vi "Instrument Manager Loop.vi"(8 "System Control":refnum<queue>, 11 "Instrument Manager":refnum<queue>) -> (0 "error out":errorcluster)   [LabVIEW 2020, in "Mock LC Parser.lvlib" / "Instrument Manager.lvlib"]
uses:
  Instrument Manager.lvlib
  support/Message Queue/Message Cluster.ctl
  Instrument State.ctl
  <vilib>/Utility/error.llb/Error Cluster From Error Code.vi
  <vilib>/ErrorRing/Error Ring.xnode
  support/Message Queue/Message Queue.lvlib
  Mock LC Parser.lvlib
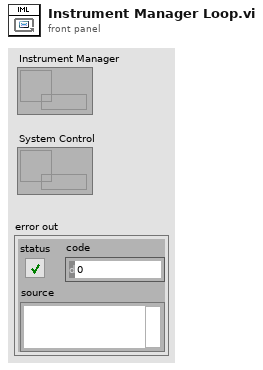
[diagram p1: front panel]
types:
  T1 = cluster{"Time Stamp":timestamp, "Peaks":string[][]}[]
  T2 = typedef "Mock LC Parser.lvlib/Instrument Manager.lvlib/Instrument State.ctl" = cluster{"Data Directory":path, "Last Report Number":i32, "Yield":dbl, "Max Concentration (mM)":dbl, "Report File Pattern":string, "Current Data File":path, "Peak Data Array":cluster{"Time Stamp":timestamp, "Peaks":string[][]}[], "Average Peak Data":cluster{"Time Stamp":timestamp, "Peaks":string[][]}, "Points to Average":i32}
  T3 = cluster{"seconds since 1Jan1904":timestamp, "Peaks":string[][]}
  T4 = cluster{"seconds since 1Jan1904":timestamp, "Peaks":string[][]}[]
  T5 = cluster{"Time Stamp":timestamp, "Peaks":string[][]}
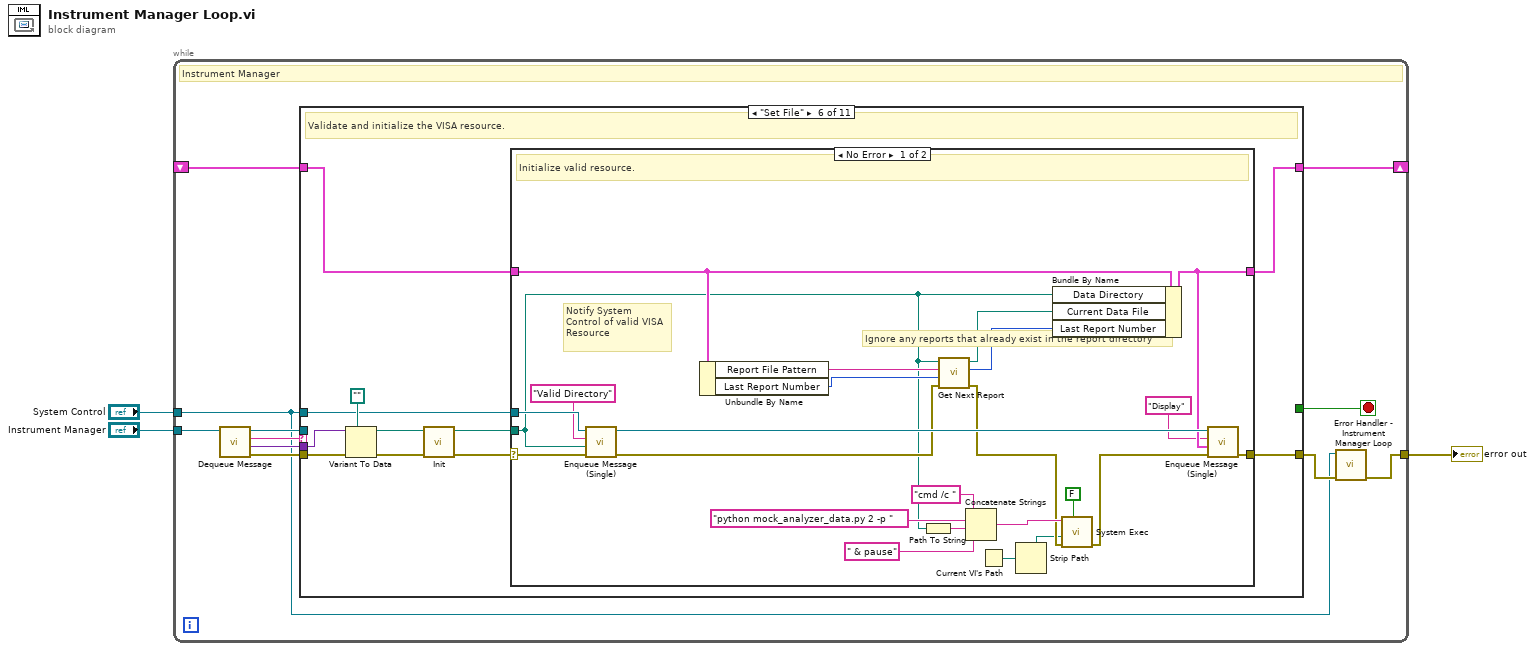
[diagram p0: block diagram]
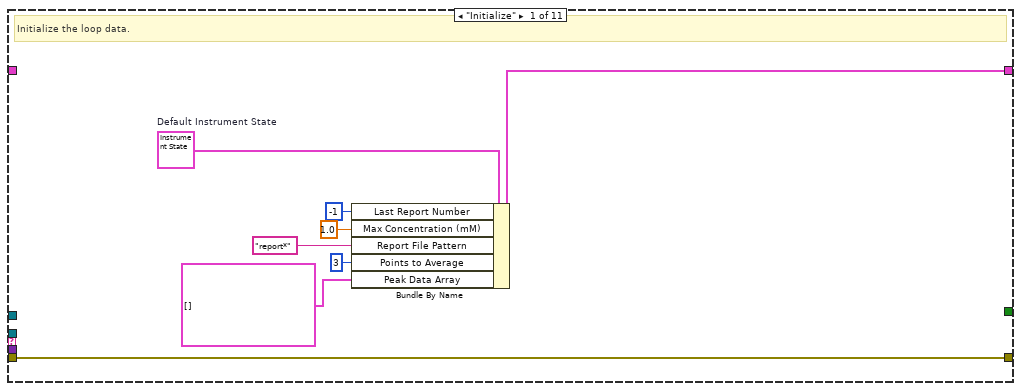
[diagram p2: hidden frame]
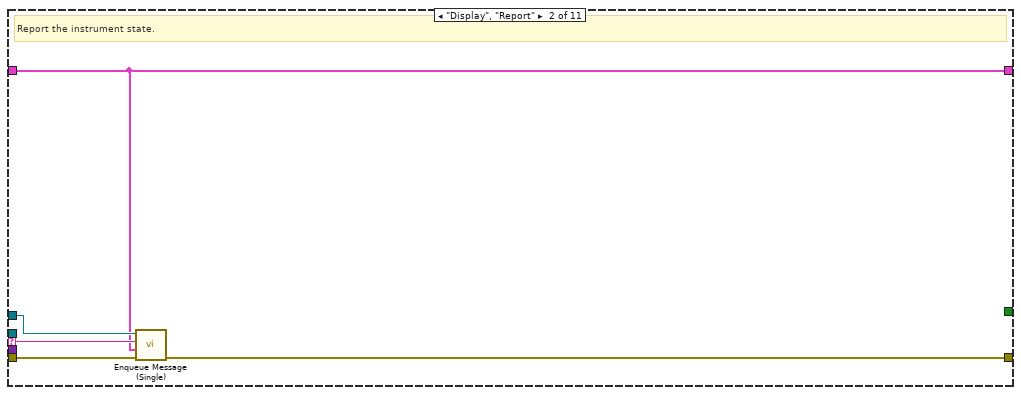
[diagram p3: hidden frame]
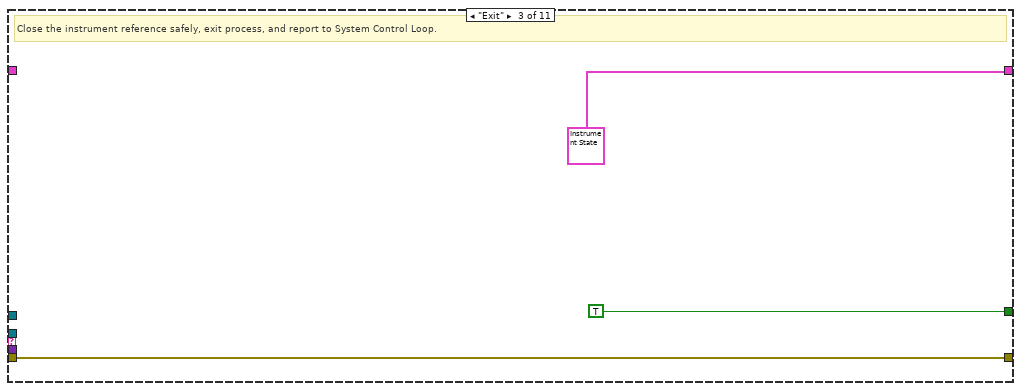
[diagram p4: hidden frame]
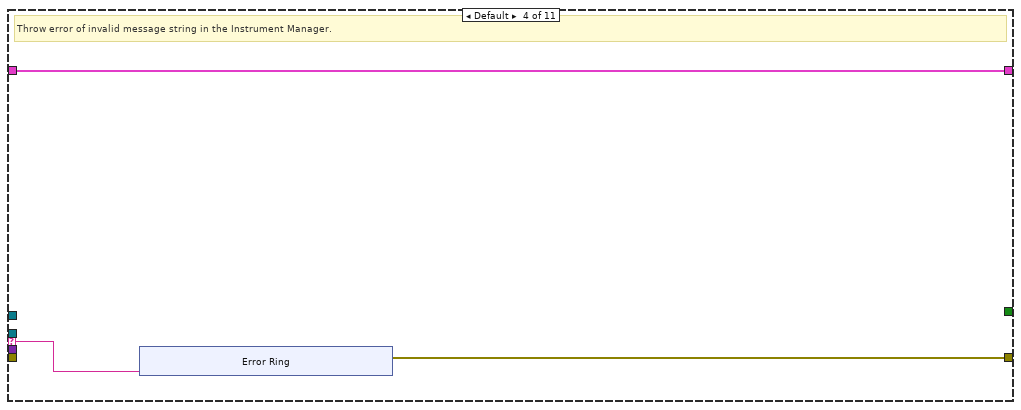
[diagram p5: hidden frame]
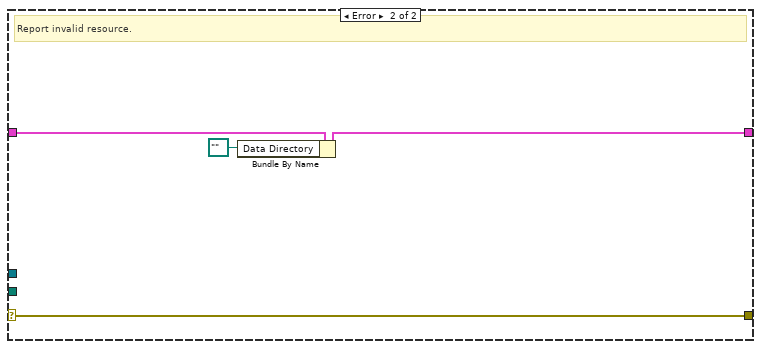
[diagram p7: hidden frame]
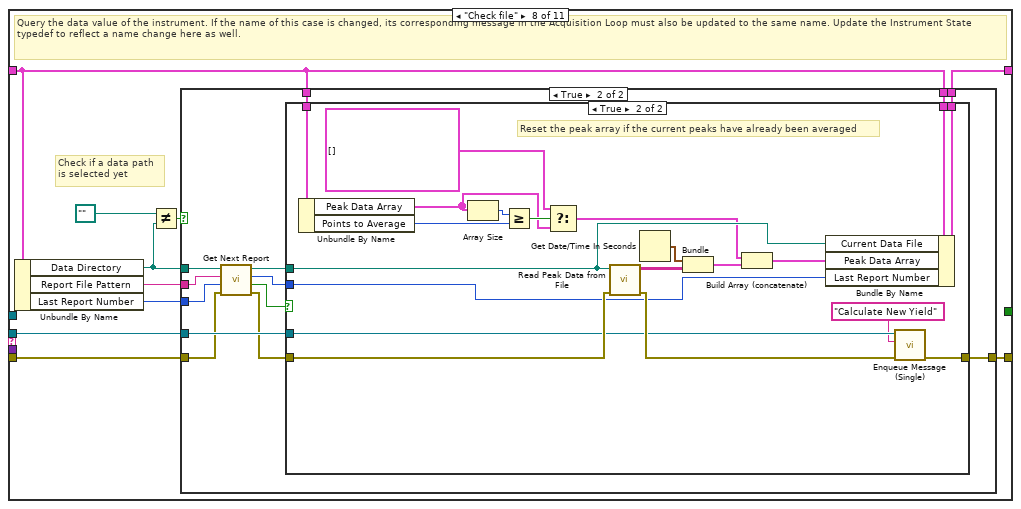
[diagram p9: hidden frame]
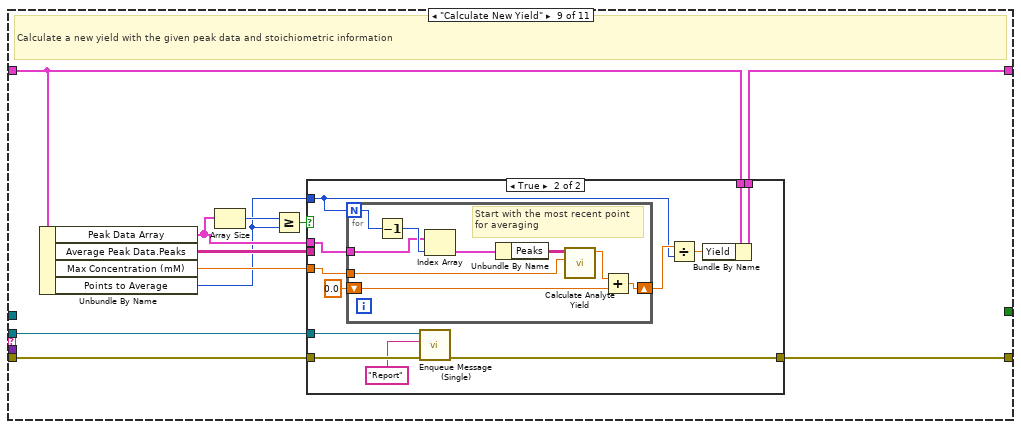
[diagram p12: hidden frame]
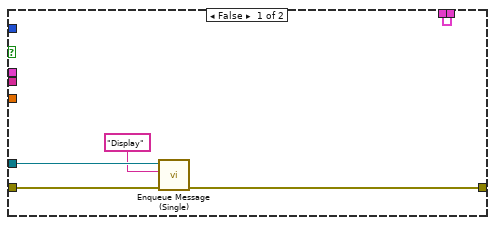
[diagram p13: hidden frame]
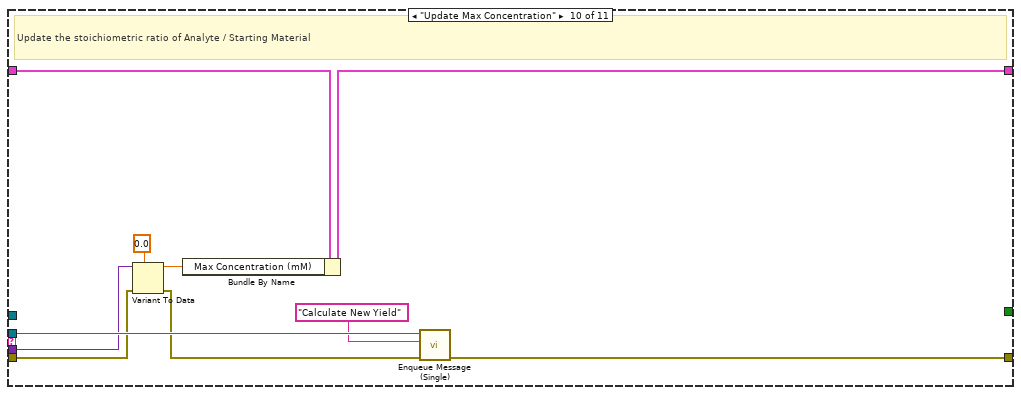
[diagram p14: hidden frame]
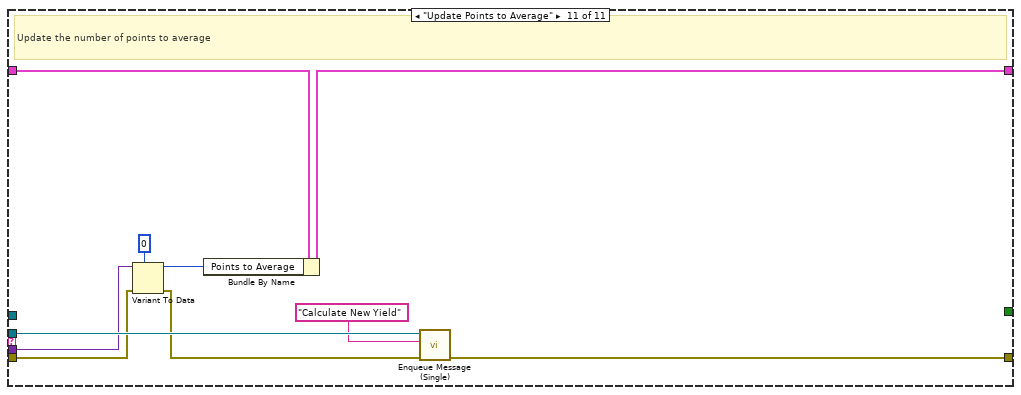
[diagram p15: hidden frame]
diagram:
  n1 = while {
    tunnel: "Instrument Manager" -> [w14]
    tunnel: "System Control" -> [w4]
    tunnel: [w8] -> w1
    shift-right: [w6] -> _
    shift-left: _ -> [w7]
    stop <- w5 stop-if-true
    # "Instrument Manager"
    n2 = call "Dequeue Message.vi"("Message Queue"=w14) -> ("error out"=w10:errorcluster, "Message Data"=w11:variant, "Message"=w13:string, "dup Message Queue"=w12:refnum<queue>)  [unwired: 7 in]
    n3 = case shown="\"Set File\"" w13 {
      selector: w13 -> [_ w25 _ w32 _ _ _ _ _ _ _]
      tunnel: w12 -> [_ _ _ _ _ _ _ w87 w137 w174 w184]
      tunnel: w4 -> [_ w26 _ _ _ w43 _ _ _ _ _]
      tunnel: w11 -> [_ _ _ _ _ w50 _ _ _ w170 w180]
      tunnel: w10 -> [w21 w27 w28 _ w41 w49 w83 w92 w139 w172 w182]
      tunnel: [w21 w23 w28 w31 w41 w53 w83 w88 w138 w175 w185] -> w9
      tunnel: w7 -> [_ w24 _ w33 w42 w52 w82 w85 w140 w176 w186]
      tunnel: [w20 w24 T2 {"Data Directory"=path "", "Last Report Number"=0, "Yield"=0.0, "Max Concentration (mM)"=1.0, "Report File Pattern"="", "Current Data File"=path "", "Peak Data Array"=[], "Average Peak Data"={"Time Stamp"=timestamp(0 s since 1904-01-01), "Peaks"=[]}, "Points to Average"=3} w33 w42 w51 w82 w93 w141 w177 w187] -> w6
      tunnel: [_ _ TRUE _ _ _ _ _ _ _ _] -> w5
      frame "Initialize" {
        w22 = T2 {"Data Directory"=path "", "Last Report Number"=0, "Yield"=0.0, "Max Concentration (mM)"=1.0, "Report File Pattern"="", "Current Data File"=path "", "Peak Data Array"=[], "Average Peak Data"={"Time Stamp"=timestamp(0 s since 1904-01-01), "Peaks"=[]}, "Points to Average"=3}  # Default Instrument State
        # "Initialize the loop data."
        n4 = Bundle By Name(cluster=w22, "Last Report Number"=-1, "Max Concentration (mM)"=1.0 ("Stoichiometry"), "Report File Pattern"="report*", "Points to Average"=3, "Peak Data Array"=T1 []) -> (w20:T2)
      }
      frame "Display", "Report" {
        # "Report the instrument state."
        n5 = call "Enqueue Message (Single).vi"("error in (no error)"=w27, "Message Data"=w24, "Message"=w25, "Message Queue"=w26) -> ("error out"=w23:errorcluster)  [unwired: 6 in, 1 out]
      }
      frame "Exit" {
        # "Close the instrument reference safely, exit process, and report to System Control Loop."
      }
      frame Default {
        # "Throw error of invalid message string in the Instrument Manager."
        n6 = xnode "Error Ring"("parameter 0"=w32) -> ("error out"=w31:errorcluster)
      }
      frame "--- Copy This Frame ---" {
        # "Copy this frame and add responses to instrument specific messages."
      }
      frame "Set File" {
        # "Validate and initialize the VISA resource."
        n7 = Variant To Data(error in=w49, type=path "", Variant=w50) -> (data=w47:path, error out=w48:errorcluster)
        n8 = call "Init.vi"("error in (no error)"=w48, "VISA resource in"=w47) -> ("error out"=w44:errorcluster, "Data Output File Out"=w45:path)  [unwired: 8 in]
        n9 = case shown="No Error" w44 {
          selector: w44 -> [w77 w79]
          tunnel: w45 -> [w57 _]
          tunnel: [w67 w79] -> w53
          tunnel: w52 -> [w74 w81]
          tunnel: [w66 w80] -> w51
          tunnel: w43 -> [w76 _]
          frame No Error {
            # "Ignore any reports that already exist in the report directory"
            # "Notify System Control of valid VISA Resource"
            # "Initialize valid resource."
            n10 = call "Enqueue Message (Single).vi"("error in (no error)"=w77, "Message Data"=w57, "Message"="Valid Directory", "Message Queue"=w76) -> ("error out"=w69:errorcluster, "dup Message Queue"=w70:refnum<queue>)  [unwired: 6 in]
            n11 = Unbundle By Name(w74) -> ("Report File Pattern"=w73:string, "Last Report Number"=w72:i32)
            n12 = Path To String(path=w57) -> (string=w60:string)
            n13 = call "Get Next Report.vi"("error in"=w69, "Last Report Number (-1)"=w72, "Report File Pattern"=w73, "Data Directory"=w57) -> ("error out"=w59:errorcluster, "Report number"=w71:i32, "Report Path"=w68:path)  [unwired: 4 in, 1 out]
            n14 = Concatenate Strings("cmd /c " ("string"), "python mock_analyzer_data.py 2 -p " ("string"), w60, " & pause" ("string")) -> (w64:string)
            n15 = Current VI's Path() -> (path=w55:path)
            n16 = Strip Path(path=w55) -> (stripped path=w54:path)  [unwired: 1 out]
            n17 = Bundle By Name(cluster=w74, "Data Directory"=w57, "Current Data File"=w68, "Last Report Number"=w71) -> (w66:T2)
            n18 = call <vilib>:"System Exec.vi"("wait until completion? (T)"=FALSE, "error in (no error)"=w59, "working directory"=w54, "command line"=w64) -> ("error out"=w58:errorcluster)  [unwired: 4 in, 3 out]
            n19 = call "Enqueue Message (Single).vi"("error in (no error)"=w58, "Message Data"=w66, "Message"="Display", "Message Queue"=w70) -> ("error out"=w67:errorcluster)  [unwired: 6 in, 1 out]
          }
          frame Error {
            # "Report invalid resource."
            n20 = Bundle By Name(cluster=w81, "Data Directory"=path "" ("Data File")) -> (w80:T2)
          }
        }
      }
      frame "--- Copy for Get State Messages ---" {
        # "#CodeNeeded - Use the Bundle by Name function to bundle the new state value into the Instrument State cluster."
        # "#CodeNeeded - Add instrument driver call to query the instrument state requested"
        # "Duplicate this case for messages cases that will query the instrument state."
      }
      frame "Check file" {
        # "Check if a data path\nis selected yet"
        # "Query the data value of the instrument. If the name of this case is changed, its corresponding message in the Acquisition Loop must also be updated to the same name. Update the Instrument State typedef to reflect a name change here as well."
        n21 = Unbundle By Name(w85) -> ("Data Directory"=w91:path, "Report File Pattern"=w86:string, "Last Report Number"=w84:i32)
        n22 = Not Equal?(x=path "", y=w91) -> (x != y?=w89:bool)
        n23 = case shown="True" w89 {
          tunnel: [w94 w105] -> w93
          tunnel: w91 -> [_ w101]
          tunnel: w92 -> [w95 w97]
          tunnel: w86 -> [_ w99]
          tunnel: [w95 w108] -> w88
          tunnel: w87 -> [_ w107]
          tunnel: w85 -> [w94 w106]
          tunnel: w85 -> [_ w100]
          tunnel: w84 -> [_ w98]
          frame False {
            # "Do nothing if no directory is selected"
          }
          frame True {
            n24 = call "Get Next Report.vi"("error in"=w97, "Last Report Number (-1)"=w98, "Report File Pattern"=w99, "Data Directory"=w101) -> ("error out"=w96:errorcluster, "New report?"=w104:bool, "Report number"=w102:i32, "Report Path"=w103:path)  [unwired: 4 in]
            n25 = case shown="True" w104 {
              tunnel: w103 -> [_ w120]
              tunnel: w96 -> [w110 w130]
              tunnel: [w110 w128] -> w108
              tunnel: w107 -> [_ w127]
              tunnel: w106 -> [w109 w123]
              tunnel: [w109 w122] -> w105
              tunnel: w102 -> [_ w121]
              tunnel: w100 -> [_ w118]
              frame False {
              }
              frame True {
                # "Reset the peak array if the current peaks have already been averaged"
                n26 = Unbundle By Name(w118) -> ("Peak Data Array"=w114:T1, "Points to Average"=w111:i32)
                n27 = Array Size(array=w114) -> (size(s)=w116:i32)
                n28 = Greater Or Equal?(x=w116, y=w111) -> (x >= y?=w115:bool)
                n29 = Select(t=T1 [] ("Peak Data Array"), s=w115, f=w114) -> (s? t:f=w112:T1)
                n30 = call "Read Peak Data from File.vi"("error in (no error)"=w130, "Data File"=w120) -> ("error out"=w129:errorcluster, "Peaks"=w124:string[][])  [unwired: 8 in]
                n31 = Get Date/Time In Seconds() -> (seconds since 1Jan1904=w125:timestamp)
                n32 = Bundle("seconds since 1Jan1904"=w125, "Peaks"=w124) -> (w119:T3)  [unwired: 1 in]
                n33 = Build Array (concatenate)(w112, w119) -> (w117:T4)
                n34 = Bundle By Name(cluster=w123, "Current Data File"=w120, "Peak Data Array"=w117, "Last Report Number"=w121) -> (w122:T2)
                n35 = call "Enqueue Message (Single).vi"("error in (no error)"=w129, "Message"="Calculate New Yield", "Message Queue"=w127) -> ("error out"=w128:errorcluster)  [unwired: 7 in, 1 out]
              }
            }
          }
        }
      }
      frame "Calculate New Yield" {
        # "Calculate a new yield with the given peak data and stoichiometric information"
        n36 = Unbundle By Name(w140) -> ("Peak Data Array"=w133:T1, "Average Peak Data.Peaks"=w134:string[][], "Max Concentration (mM)"=w136:dbl, "Points to Average"=w131:i32)
        n37 = Array Size(array=w133) -> (size(s)=w132:i32)
        n38 = Greater Or Equal?(x=w132, y=w131) -> (x >= y?=w135:bool)
        n39 = case shown="True" w135 {
          tunnel: [w146 w158] -> w141
          tunnel: w140 -> [w146 w157]
          tunnel: w139 -> [w145 w156]
          tunnel: [w144 w147] -> w138
          tunnel: w137 -> [w143 w155]
          tunnel: w136 -> [_ w153]
          tunnel: w134 -> [_ _]
          tunnel: w133 -> [_ w152]
          tunnel: w131 -> [_ w148]
          frame False {
            n40 = call "Enqueue Message (Single).vi"("error in (no error)"=w145, "Message"="Display", "Message Queue"=w143) -> ("error out"=w144:errorcluster)  [unwired: 7 in, 1 out]
          }
          frame True {
            n41 = for {
              N: w148 -> [w162]
              tunnel: w153 -> [w167]
              tunnel: w152 -> [w160]
              shift-right: [w163] -> w150
              shift-left: 0.0 -> [w165]
              # "Start with the most recent point\nfor averaging"
              n42 = Decrement(x=w162) -> (x-1=w161:i32)
              n43 = Index Array(array=w160, index=w161) -> (element=w159:T5)
              n44 = Unbundle By Name(w159) -> ("Peaks"=w166:string[][])
              n45 = call "Calculate Analyte Yield.vi"("Max Concentration"=w167, "Peaks"=w166) -> ("Yield out"=w164:dbl)  [unwired: 9 in]
              n46 = Add(x=w164, y=w165) -> (x+y=w163:dbl)
            }
            n47 = call "Enqueue Message (Single).vi"("error in (no error)"=w156, "Message"="Report", "Message Queue"=w155) -> ("error out"=w147:errorcluster)  [unwired: 7 in, 1 out]
            n48 = Divide(x=w150, y=w148) -> (x/y=w149:dbl)
            n49 = Bundle By Name(cluster=w157, "Yield"=w149) -> (w158:T2)
          }
        }
      }
      frame "Update Max Concentration" {
        # "Update the stoichiometric ratio of Analyte / Starting Material"
        n50 = Variant To Data(error in=w172, type=0.0, Variant=w170) -> (data=w168:dbl, error out=w171:errorcluster)
        n51 = Bundle By Name(cluster=w176, "Max Concentration (mM)"=w168) -> (w177:T2)
        n52 = call "Enqueue Message (Single).vi"("error in (no error)"=w171, "Message"="Calculate New Yield", "Message Queue"=w174) -> ("error out"=w175:errorcluster)  [unwired: 7 in, 1 out]
      }
      frame "Update Points to Average" {
        # "Update the number of points to average"
        n53 = Variant To Data(error in=w182, type=0, Variant=w180) -> (data=w178:i32, error out=w181:errorcluster)
        n54 = Bundle By Name(cluster=w186, "Points to Average"=w178) -> (w187:T2)
        n55 = call "Enqueue Message (Single).vi"("error in (no error)"=w181, "Message"="Calculate New Yield", "Message Queue"=w184) -> ("error out"=w185:errorcluster)  [unwired: 7 in, 1 out]
      }
    }
    n56 = call "Error Handler - Instrument Manager Loop.vi"("error in (no error)"=w9, "Message Queue"=w4) -> ("dup error in"=w8:errorcluster)  [unwired: 8 in, 1 out]
  }
  "error out" <- w1
